vi "Close Some Modal Running VIs.vi"() -> ()   [LabVIEW 2019]
doc: "Utility to close a modal VI when it has been brought to the foreground and reserved to run. This locks up LabVIEW so this VI will present a list of VIs to optionally close.\nScott Hannahs, National High Magnetic Field Lab\nJanuary 2005\n<sth@magnet.fsu.edu>"
panel:
  in  "OK Button":bool
  in  "VIs to close":i32[](listbox)
  out "Slide":i32(slide) scale=0.0..50.0
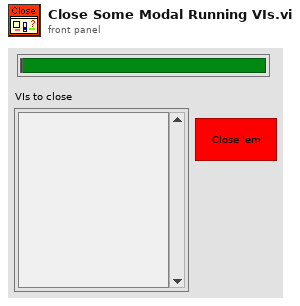
[diagram p1: front panel]
types:
  T1 = enum32{"Bad", "Idle", "Run top level", "Running"}
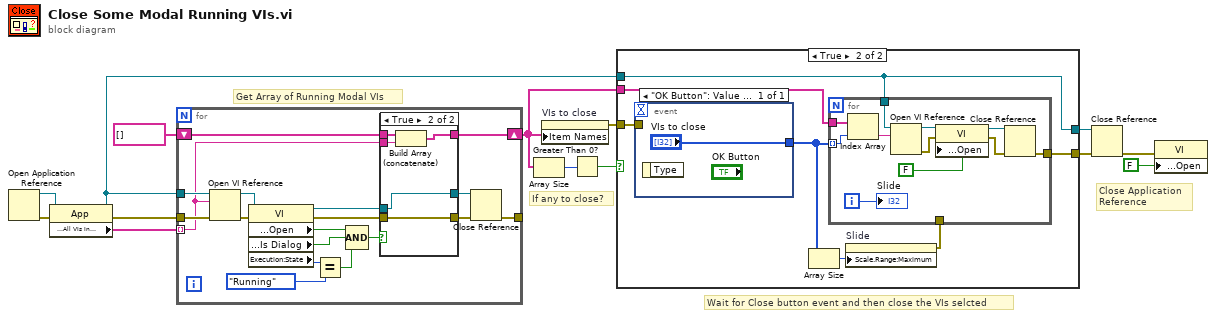
[diagram p0: block diagram]
diagram:
  # "If any to close?"
  # "Close Application\nReference"
  # "Wait for Close button event and then close the VIs selcted"
  # "Get Array of Running Modal VIs"
  n1 = Open Application Reference() -> (0:w14:errorcluster, 3:w13:refnum<vi>)  [unwired: 4 in]
  n2 = property class="App"(reference=w13, error in=w14) -> (reference out=w2:refnum<vi>, error out=w12:errorcluster, "Application:All VIs In Memory"=w11:string[])
  n3 = for {
    tunnel: w12 -> [w32]
    tunnel: w11 -> [w16] mode=indexing
    tunnel: w2 -> [w17]
    tunnel: [w21] -> _
    shift-right: [w15] -> w5
    shift-left: string[] [] -> [w18]
    n4 = Open VI Reference(application reference (local)=w17, vi path=w16, error in (no error)=w32) -> (vi reference=w30:refnum<vi>, error out=w31:errorcluster)  [unwired: 3 in]
    n5 = property class="VI"(reference=w30, error in=w31) -> (reference out=w24:refnum<vi>, error out=w25:errorcluster, "Front Panel Window:Open"=w27:bool, "Front Panel Window:Is Dialog"=w28:bool, "Execution:State"=w29:T1)
    n6 = Equal?(x=w29, y=T1."Running") -> (x = y?=w19:bool)
    n7 = Compound Arithmetic op=AND(w27, w28, w19) -> (w26:bool)
    n8 = case shown="True" w26 {
      tunnel: w25 -> [w34 w38]
      tunnel: w24 -> [w35 w36]
      tunnel: [w34 w38] -> w23
      tunnel: [w35 w36] -> w22
      tunnel: w18 -> [w33 w40]
      tunnel: w16 -> [_ w39]
      tunnel: [w33 w37] -> w15
      frame False {
      }
      frame True {
        n9 = Build Array (concatenate)(w40, w39) -> (w37:string[])
      }
    }
    n10 = Close Reference(reference=w22, error in (no error)=w23) -> (error out=w21:errorcluster)
  }
  n11 = Array Size(array=w5) -> (size(s)=w4:i32)
  n12 = property on="VIs to close" class="LstBox (strict)"("Item Names"=w5) -> (error out=w7:errorcluster)  [unwired: 2 in, 1 out]
  n13 = Greater Than 0?(x=w4) -> (x > 0?=w3:bool)
  n14 = case shown="True" w3 {
    tunnel: w7 -> [w42 w48]
    tunnel: [w42 w45] -> w6
    tunnel: w5 -> [_ w44]
    tunnel: w2 -> [w41 w43]
    tunnel: [w41 w43] -> w1
    frame False {
    }
    frame True {
      n15 = event shown="[0] \"OK Button\": Value Change" {
        selector: _ -> [_]
        dyn-events: _ -> [_]
        timeout: _ -> [_]
        tunnel: w48 -> [_]
        tunnel: ["VIs to close"] -> w47
        event "OK Button": Value Change {
          n16 = event-data() -> ()  [unwired: 1 in, 1 out]
        }
      }
      n17 = Array Size(array=w47) -> (size(s)=w49:i32)
      n18 = property on="Slide" class="Slide (strict)"("Scale.Range:Maximum"=w49) -> (error out=w46:errorcluster)  [unwired: 2 in, 1 out]
      n19 = for {
        tunnel: w47 -> [w57] mode=indexing
        tunnel: w46 -> [_]
        tunnel: w44 -> [w58]
        tunnel: w43 -> [w51]
        tunnel: [w50] -> w45
        i -> [w60]
        n20 = Index Array(array=w58, index=w57) -> (element=w59:string)
        n21 = Open VI Reference(application reference (local)=w51, vi path=w59) -> (vi reference=w56:refnum<vi>, error out=w55:errorcluster)  [unwired: 4 in]
        n22 = property class="VI"(reference=w56, error in=w55, "Front Panel Window:Open"=FALSE) -> (reference out=w53:refnum<vi>, error out=w52:errorcluster)
        n23 = Close Reference(reference=w53, error in (no error)=w52) -> (error out=w50:errorcluster)
        "Slide" <- w60
      }
    }
  }
  n24 = Close Reference(reference=w1, error in (no error)=w6) -> (error out=w10:errorcluster)
  n25 = property class="VI"(error in=w10, "Front Panel Window:Open"=FALSE) -> ()  [unwired: 1 in, 2 out]
